vi "LightSheet_Example_IMAQ.vi"() -> ()   [LabVIEW 2019]
doc: "This example is similar to the simple example, but uses get/set line timeing for controlling the exposure.\nExposureTime = LineTime * ExposureLines\nBeside of the line timing part, a simple recording of an image sequence and the image access afterwards is done.\nIt is a good starting point for writing own applications, especially for light sheet application development.\nBut it will not be fail save, i.e. doesnt react on errors, just handles them forward to the end\n\nUsage:\nSelect your required image count and the required line tiime + number of exposure lines before you start the program.\nOnce started, the camera class will be initialized and images will be recorded automatically.\nWhen acquisition has finished you can address the images and set a certain roi \nTo finish the program click on quit application, this will force fan exit of the camera class"
uses:
  camera/Camera.lvclass
  pco.sdk/SpecialCommandsEdge/SpecialCommandsEdge.lvlib
panel:
  in  "dwExposureLines":u32=100
  in  "wTimeBase":u16(ring)=1 items=["ns", "us", "ms"]
  in  "dwLineTime":u32=50
  out "rawImage":u16[][](array[numeric])
  out "Image":T1(plugin-control)
  in  "data_format":T2(ring)=enum."Mono16"
  in  "Image Index":u32 max=99
  out "Recorded Images":u32
  in  "Quit":bool
  in  "cropY1":u64=2 min=2 max=1040 step=1
  in  "cropX1":u64=2 min=2 max=1392 step=1
  in  "cropY0":u64=1 min=1 max=1039 step=1
  in  "cropX0":u64=1 min=1 max=1391 step=1
  out "Image Height":u64
  out "Image Width":u64
  in  "dwImgCount":u32=10 caption="Required Number of Images" max=4023
  out "Error":errorcluster {"code" format="%x"}
  # "This example is similar to the simple example, but uses get/set line timeing for controlling the exposure.\nExposureTime = LineTime * ExposureLines\nBeside of the line timing part, a simple recording of an image sequence and the image access afterwards is done.\nIt is a good starting point for writing own applications, especially  for light sheet application development.\nBut it will not be fail save, i.e. doesnt react on errors, just handles them forward to the end\n\nUsage:\nSelect your required image count and the required line tiime + number of exposure lines before you start the program.\nOnce started, the camera class will be initialized and images will be recorded automatically.\nWhen acquisition has finished you can address the images and set a certain roi \nTo finish the program click on quit application, this will force fan exit of the camera class"
  # "pco.labview"
  # "Camera Setup"
  # "Recording Control"
  # "Parameters for image readout"
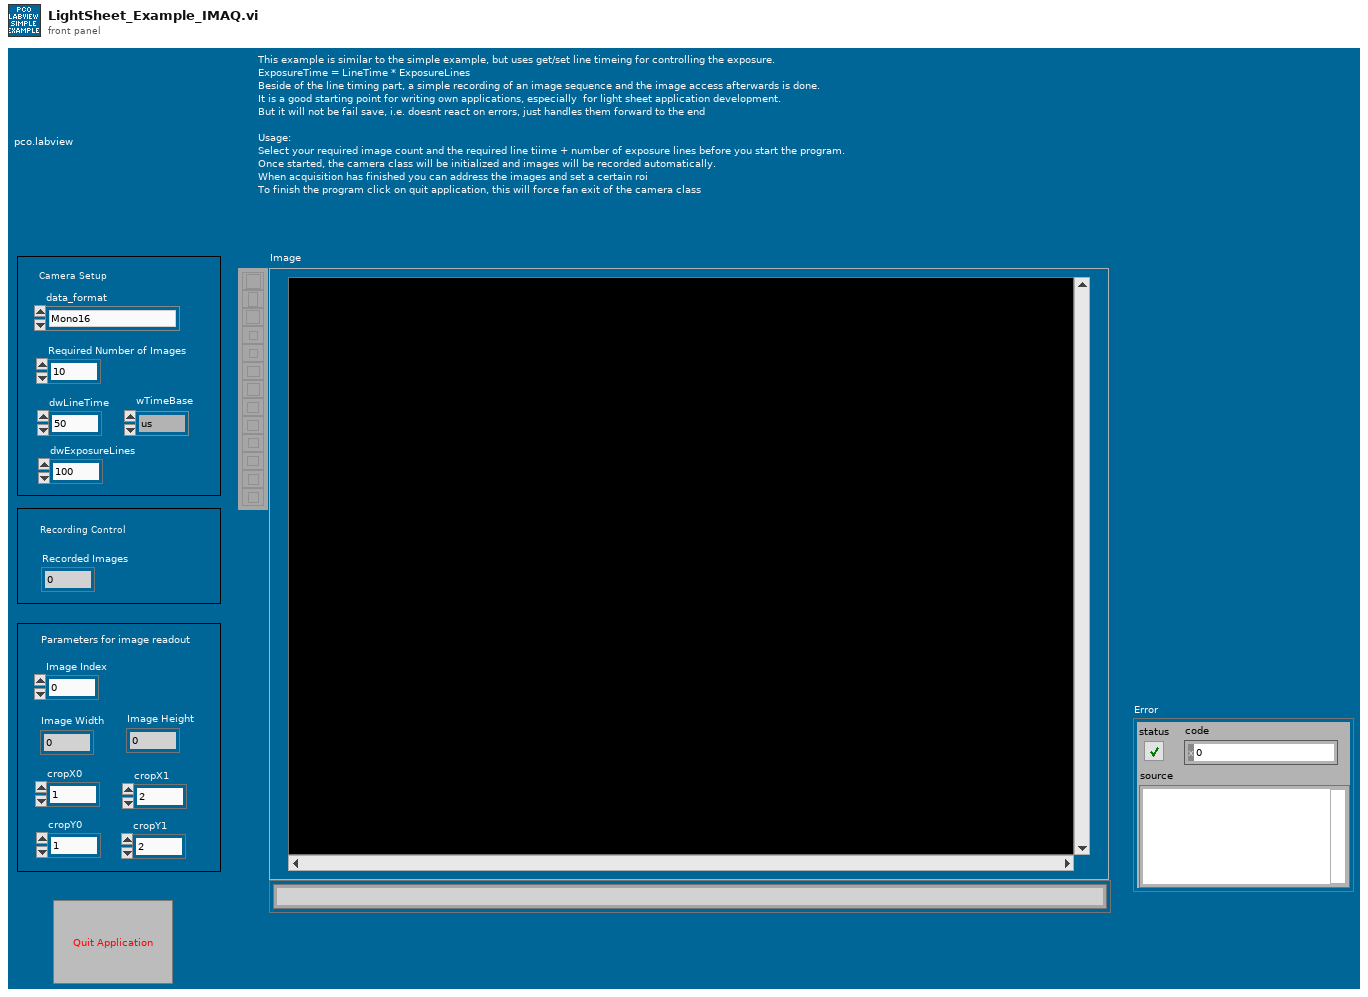
[diagram p1: front panel]
types:
  T1 = typedef "IMAQ Image.ctl" = refnum<image>
  T2 = enum16{"Undefined", "Mono8", "Mono16", "BGRA8", "RGBA8", "BGRA16", "RGBA16", "CompressedMono8"}
  T3 = enum8{"Enabled", "Disabled", "Disabled and Grayed Out"}
  T4 = enum16{"sequence", "sequence non blocking", "ring buffer", "fifo", "tif", "multitif", "pcoraw", "b16", "dicom", "multidicom", "camram_ring", "camram_segment"}
  T5 = cluster{"serial":u32, "type":u16, "sub_type":u16, "interface_type":u16, "bit_resolution":u16, "min_exposure_time_s":dbl, "max_exposure_time_s":dbl, "min_exposure_step_s":dbl, "min_delay_time_s":dbl, "max_delay_time_s":dbl, "min_delay_step_s":dbl, "min_width":u64, "min_height":u64, "max_width":u64, "max_height":u64, "roi_step_horz":u64, "roi_step_vert":u64, "roi_symmetric_horz":bool, "roi_symmetric_vert":bool, "has_timestamp_mode":bool, "has_timestamp_mode_ascii_only":bool, "pixelrate_vec":u32[], "conversion_factor_vec":sgl[], "has_trigger_mode_extexpctrl":bool, "has_acquire_mode":bool, "has_ext_acquire_mode":bool, "has_metadata_mode":bool, "has_ram":bool, "binning_horz_vec":u16[], "binning_vert_vec":u16[], "has_average_binning":bool, "pixel_format_vec":u32[]}
  T6 = typedef "Image Type" = u32
  T7 = typedef "Camera.lvclass/binning.ctl" = cluster{"vert":u16, "horz":u16, "mode":u16}
  T8 = cluster{"exposure_time_s":dbl, "delay_time_s":dbl, "roi":cluster{"x0":u64, "y0":u64, "x1":u64, "y1":u64}, "timestamp_mode":u16, "pixelrate":u32, "conversion_factor":sgl, "trigger_mode":u16, "acquire_mode":u16, "acquire_sequence_number":u32, "metadata_mode":u16, "noisefilter_mode":u16, "pixel_format":u32, "binning":T7, "auto_exposure":cluster{"region":u16, "min_exposure_s":dbl, "max_exposure_s":dbl}}
  T9 = cluster{"Plane 4 (alpha)":u16, "Plane 1 (Red)":u16, "Plane 2 (Green)":u16, "Plane 3 (Blue)":u16}[][]
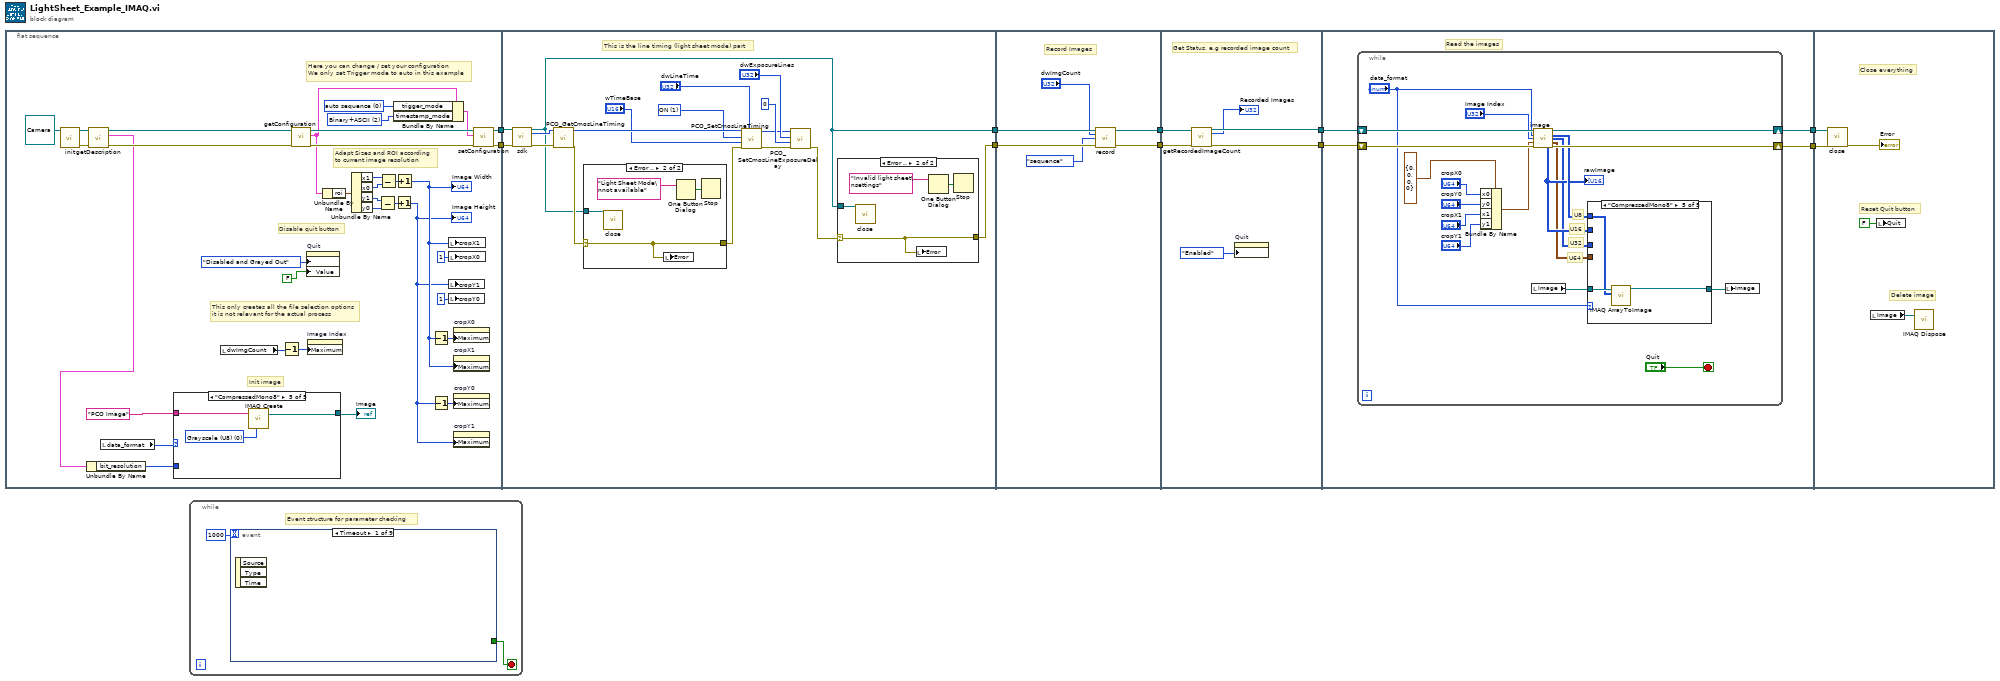
[diagram p0: block diagram]
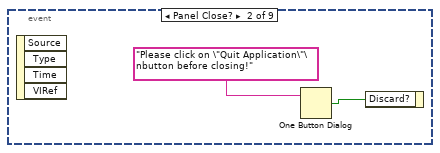
[diagram p2: hidden frame]
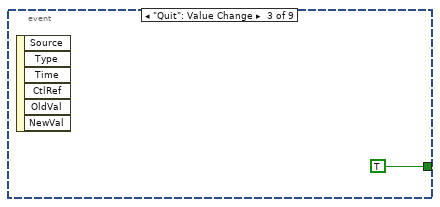
[diagram p3: hidden frame]
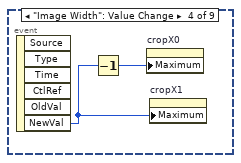
[diagram p4: hidden frame]
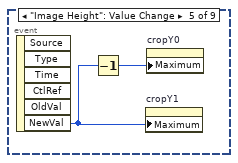
[diagram p5: hidden frame]
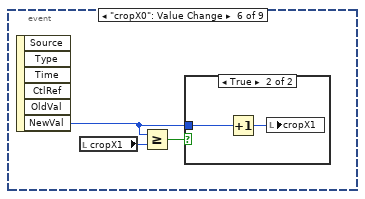
[diagram p6: hidden frame]
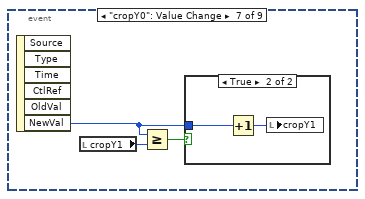
[diagram p8: hidden frame]
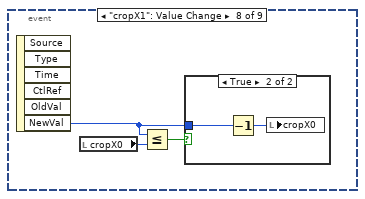
[diagram p10: hidden frame]
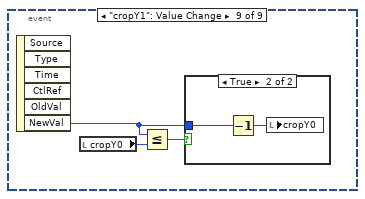
[diagram p12: hidden frame]
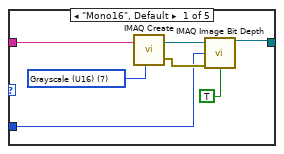
[diagram p14: hidden frame]
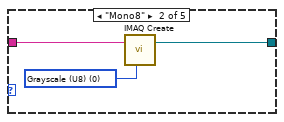
[diagram p15: hidden frame]
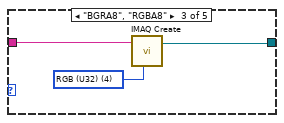
[diagram p16: hidden frame]
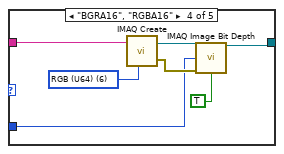
[diagram p17: hidden frame]
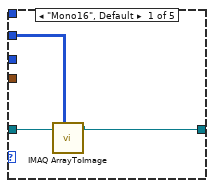
[diagram p20: hidden frame]
diagram:
  n1 = flat-sequence {
    tunnel: [w40] -> w4
    tunnel: [w39] -> w2
    tunnel: w4 -> [w81]
    tunnel: [w69] -> w3
    tunnel: w2 -> [w80]
    tunnel: [w70] -> w1
    tunnel: w3 -> [w101]
    tunnel: w1 -> [w100]
    tunnel: [w98] -> w10
    tunnel: [w97] -> w9
    tunnel: w10 -> [w107]
    tunnel: w9 -> [w106]
    tunnel: [w105] -> w8
    tunnel: [w104] -> w7
    tunnel: w8 -> [w110]
    tunnel: w7 -> [w111]
    tunnel: [w109] -> w6
    tunnel: [w108] -> w5
    tunnel: w6 -> [w148]
    tunnel: w5 -> [w147]
    frame #0 {
      w24 = u16 2 items=["OFF", "Binary", "Binary+ASCII", "ASCII"] ("TimestampMode")
      w44 = u16 0 items=["auto sequence"=0, "software trigger"=1, "external exposure start & software trigger"=2, "external exposure control"=3, "external synchronized"=4, "fast external exposure control"=5, "external CDS control"=6, "slow external exposure control"=7, "external synchronized HDSDI"=258] ("TriggerMode")
      # "Init image"
      # "This only creates all the file selection options\nit is not relevant for the actual process"
      # "Adapt Sizes and ROI according\nto current image resolution"
      # "Disable quit button"
      # "Here you can change / set your configuration\nWe only set Trigger mode to auto in this example"
      n2 = call-dynamic "init.vi"("Camera in"=refnum<class "Camera.lvclass"> refnum ("PCOCamera in")) -> ("Camera out"=w15:refnum<class "Camera.lvclass">, "error out"=w16:errorcluster)  [unwired: 8 in]
      n3 = call-dynamic "getDescription.vi"("error in (no error)"=w16, "Camera in"=w15) -> ("error out"=w13:errorcluster, "description"=w12:T5, "Camera out"=w14:refnum<class "Camera.lvclass">)  [unwired: 7 in]
      n4 = Unbundle By Name(w12) -> ("bit_resolution"=w11:u16)
      n5 = local read "data_format"() -> (w19:T2)
      n6 = case shown="\"CompressedMono8\"" w19 {
        tunnel: "PCO Image" ("Image Name") -> [w51 w55 w57 w64 w67]
        tunnel: [w47 w53 w56 w61 w66] -> w18
        tunnel: w11 -> [w46 _ _ w59 _]
        frame "Mono16", Default {
          w52 = T6 7 items=["Grayscale (U8)", "Grayscale (I16)", "Grayscale (SGL)", "Complex (CSG)", "RGB (U32)", "HSL (U32)", "RGB (U64)", "Grayscale (U16)"] ("Image Type")
          n7 = call "IMAQ Create"("Image Name"=w51, "Image Type"=w52) -> ("New Image"=w49:T1, "error out"=w48:errorcluster)  [unwired: 3 in]
          n8 = call "IMAQ Image Bit Depth"("Image"=w49, "Bit Depth (0)"=w46, "error in (no error)"=w48, "Get/Set Bit Depth? (Set)"=TRUE) -> ("Image Out"=w47:T1)  [unwired: 9 in, 2 out]
        }
        frame "Mono8" {
          w54 = T6 0 items=["Grayscale (U8)", "Grayscale (I16)", "Grayscale (SGL)", "Complex (CSG)", "RGB (U32)", "HSL (U32)", "RGB (U64)", "Grayscale (U16)"] ("Image Type")
          n9 = call "IMAQ Create"("Image Name"=w55, "Image Type"=w54) -> ("New Image"=w53:T1)  [unwired: 3 in, 1 out]
        }
        frame "BGRA8", "RGBA8" {
          w58 = T6 4 items=["Grayscale (U8)", "Grayscale (I16)", "Grayscale (SGL)", "Complex (CSG)", "RGB (U32)", "HSL (U32)", "RGB (U64)", "Grayscale (U16)"] ("Image Type")
          n10 = call "IMAQ Create"("Image Name"=w57, "Image Type"=w58) -> ("New Image"=w56:T1)  [unwired: 3 in, 1 out]
        }
        frame "BGRA16", "RGBA16" {
          w65 = T6 6 items=["Grayscale (U8)", "Grayscale (I16)", "Grayscale (SGL)", "Complex (CSG)", "RGB (U32)", "HSL (U32)", "RGB (U64)", "Grayscale (U16)"] ("Image Type")
          n11 = call "IMAQ Create"("Image Name"=w64, "Image Type"=w65) -> ("New Image"=w62:T1, "error out"=w60:errorcluster)  [unwired: 3 in]
          n12 = call "IMAQ Image Bit Depth"("Image"=w62, "Bit Depth (0)"=w59, "error in (no error)"=w60, "Get/Set Bit Depth? (Set)"=TRUE) -> ("Image Out"=w61:T1)  [unwired: 9 in, 2 out]
        }
        frame "CompressedMono8" {
          w68 = T6 0 items=["Grayscale (U8)", "Grayscale (I16)", "Grayscale (SGL)", "Complex (CSG)", "RGB (U32)", "HSL (U32)", "RGB (U64)", "Grayscale (U16)"] ("Image Type")
          n13 = call "IMAQ Create"("Image Name"=w67, "Image Type"=w68) -> ("New Image"=w66:T1)  [unwired: 3 in, 1 out]
        }
      }
      "Image" <- w18
      n14 = local read "dwImgCount"() -> (w20:u32)
      n15 = Decrement(x=w20) -> (x-1=w21:u32)
      n16 = call-dynamic "getConfiguration.vi"("error in (no error)"=w13, "Camera in"=w14) -> ("error out"=w42:errorcluster, "configuration"=w34:T8, "Camera out"=w43:refnum<class "Camera.lvclass">)  [unwired: 7 in]
      n17 = property on="Quit" class="Bool (strict)"("DisabledEnum"=T3."Disabled and Grayed Out" ("Disabled"), "Value"=FALSE ("Stop")) -> ()  [unwired: 2 in, 2 out]
      n18 = property on="Image Index" class="DigNum (strict)"("Maximum"=w21) -> ()  [unwired: 2 in, 2 out]
      n19 = Unbundle By Name(w34) -> ("roi"=w33:cluster{"x0":u64, "y0":u64, "x1":u64, "y1":u64})
      n20 = Unbundle By Name(w33) -> ("x1"=w31:u64, "x0"=w32:u64, "y1"=w29:u64, "y0"=w30:u64)
      n21 = Subtract(x=w29, y=w30) -> (x-y=w27:u64)
      n22 = Subtract(x=w31, y=w32) -> (x-y=w28:u64)
      n23 = Bundle By Name(cluster=w34, "trigger_mode"=w44, "timestamp_mode"=w24) -> (w41:T8)
      n24 = Increment(x=w27) -> (x+1=w25:u64)
      "Image Height" <- w25
      n25 = Increment(x=w28) -> (x+1=w26:u64)
      "Image Width" <- w26
      n26 = Decrement(x=w26) -> (x-1=w36:u64)
      n27 = Decrement(x=w25) -> (x-1=w35:u64)
      n28 = local write "cropX1"(w26) -> ()
      n29 = local write "cropX0"(u64 1 ("roiY0")) -> ()
      n30 = local write "cropY1"(w25) -> ()
      n31 = local write "cropY0"(u64 1 ("roiY0")) -> ()
      n32 = property on="cropX0" class="DigNum (strict)"("Maximum"=w36) -> ()  [unwired: 2 in, 2 out]
      n33 = property on="cropX1" class="DigNum (strict)"("Maximum"=w26) -> ()  [unwired: 2 in, 2 out]
      n34 = property on="cropY0" class="DigNum (strict)"("Maximum"=w35) -> ()  [unwired: 2 in, 2 out]
      n35 = property on="cropY1" class="DigNum (strict)"("Maximum"=w25) -> ()  [unwired: 2 in, 2 out]
      n36 = call-dynamic "setConfiguration.vi"("error in (no error)"=w42, "configuration"=w41, "Camera in"=w43) -> ("error out"=w39:errorcluster, "Camera out"=w40:refnum<class "Camera.lvclass">)  [unwired: 7 in]
    }
    frame #1 {
      w77 = u16 1 items=["OFF", "ON"] ("wParameter")
      # "This is the line timing (light sheet mode) part"
      n37 = call-dynamic "sdk.vi"("Camera in"=w81, "error in (no error)"=w80) -> ("Camera out"=w69:refnum<class "Camera.lvclass">, "sdk"=w79:u64, "error out"=w85:errorcluster)  [unwired: 11 in]
      n38 = call "PCO_GetCmosLineTiming.vi"("ph"=w79, "error in (no error)"=w85) -> ("ph out"=w78:u64, "error out"=w84:errorcluster)  [unwired: 10 in, 6 out]
      n39 = case shown="Error .." w84 {
        selector: w84 -> [w91 w92]
        tunnel: [w91 w92] -> w83
        tunnel: w69 -> [_ w93]
        frame No Error {
        }
        frame Error {
          n40 = call-dynamic "close.vi"("Camera in"=w93) -> ()  [unwired: 10 in, 1 out]
          n41 = local write "Error"(w92) -> ()
          n42 = One Button Dialog(message="Light Sheet Mode\nnot available") -> (true=w94:bool)  [unwired: 1 in]
          n43 = Stop(stop? (T)=w94) -> ()
        }
      }
      n44 = call "PCO_SetCmosLineTiming.vi"("dwLineTime"="dwLineTime", "error in (no error)"=w83, "wTimeBase"="wTimeBase", "wParameter"=w77, "ph"=w78) -> ("error out"=w82:errorcluster, "ph out"=w72:u64)  [unwired: 4 in, 1 out]
      n45 = call "PCO_SetCmosLineExposureDelay.vi"("error in (no error)"=w82, "dwDelayLines"=u32 0, "dwExposureLines"="dwExposureLines", "ph"=w72) -> ("error out"=w71:errorcluster)  [unwired: 5 in, 2 out]
      n46 = case shown="Error .." w71 {
        selector: w71 -> [w86 w87]
        tunnel: [w86 w87] -> w70
        tunnel: w69 -> [_ w88]
        frame No Error {
        }
        frame Error {
          n47 = call-dynamic "close.vi"("Camera in"=w88) -> ()  [unwired: 10 in, 1 out]
          n48 = local write "Error"(w87) -> ()
          n49 = One Button Dialog(message="Invalid light sheet\nsettings") -> (true=w89:bool)  [unwired: 1 in]
          n50 = Stop(stop? (T)=w89) -> ()
        }
      }
    }
    frame #2 {
      # "Record Images"
      n51 = call-dynamic "record.vi"("Camera in"=w101, "num_images"="dwImgCount", "record_mode"=T4."sequence", "error in (no error)"=w100) -> ("Camera out"=w98:refnum<class "Camera.lvclass">, "error out"=w97:errorcluster)  [unwired: 10 in]
    }
    frame #3 {
      # "Get Status, e.g recorded image count"
      n52 = call-dynamic "getRecordedImageCount.vi"("Camera in"=w107, "error in (no error)"=w106) -> ("Camera out"=w105:refnum<class "Camera.lvclass">, "recorded_image_count"=→"Recorded Images":u32, "error out"=w104:errorcluster)  [unwired: 11 in]
      n53 = property on="Quit" class="Bool (strict)"("DisabledEnum"=T3."Enabled" ("Disabled")) -> ()  [unwired: 2 in, 2 out]
    }
    frame #4 {
      # "Read the images"
      n54 = while {
        shift-right: [w128] -> w109
        shift-left: w110 -> [w130]
        shift-right: [w123] -> w108
        shift-left: w111 -> [w129]
        stop <- "Quit" stop-if-true
        # "U64"
        # "U32"
        # "U16"
        # "U8"
        n55 = Bundle By Name(cluster=cluster{"x0":u64, "y0":u64, "x1":u64, "y1":u64} {"x0"=0, "y0"=0, "x1"=0, "y1"=0} ("roi"), "x0"="cropX0", "y0"="cropY0", "x1"="cropX1", "y1"="cropY1") -> (w122:cluster{"x0":u64, "y0":u64, "x1":u64, "y1":u64})
        n56 = local read "Image"() -> (w115:T1)
        n57 = call-dynamic "image.vi"("Camera in"=w130, "data_format"="data_format", "image_index"="Image Index", "crop"=w122, "error in (no error)"=w129) -> ("Camera out"=w128:refnum<class "Camera.lvclass">, "image (U8)"=w119:u8[][], "image (U32)"=w117:u32[][], "image (U64)"=w116:T9, "raw_image (U16)"=w118:u16[][], "error out"=w123:errorcluster)  [unwired: 2 in, 3 out]
        "rawImage" <- w118
        n58 = case shown="\"CompressedMono8\"" "data_format" {
          tunnel: w115 -> [w133 w136 w139 w142 w145]
          tunnel: [w131 w134 w138 w140 w144] -> w114
          tunnel: w116 -> [_ _ _ w141 _]
          tunnel: w117 -> [_ _ w137 _ _]
          tunnel: w119 -> [_ w135 _ _ w143]
          tunnel: w118 -> [w132 _ _ _ _]
          frame "Mono16", Default {
            n59 = call "IMAQ ArrayToImage"("Image Pixels (U16)"=w132, "Image"=w133) -> ("Image Out"=w131:T1)  [unwired: 8 in, 1 out]
          }
          frame "Mono8" {
            n60 = call "IMAQ ArrayToImage"("Image Pixels (U8)"=w135, "Image"=w136) -> ("Image Out"=w134:T1)  [unwired: 8 in, 1 out]
          }
          frame "BGRA8", "RGBA8" {
            n61 = call "IMAQ ArrayToColorImage"("Image Pixels (U32)"=w137, "Image"=w139) -> ("Image Out"=w138:T1)  [unwired: 3 in, 1 out]
          }
          frame "BGRA16", "RGBA16" {
            n62 = call "IMAQ ArrayToColorImage"("Image"=w142, "Image Pixels (U64)"=w141) -> ("Image Out"=w140:T1)  [unwired: 3 in, 1 out]
          }
          frame "CompressedMono8" {
            n63 = call "IMAQ ArrayToImage"("Image Pixels (U8)"=w143, "Image"=w145) -> ("Image Out"=w144:T1)  [unwired: 8 in, 1 out]
          }
        }
        n64 = local write "Image"(w114) -> ()
      }
    }
    frame #5 {
      # "Delete image"
      # "Reset Quit button"
      # "Close everything"
      n65 = call-dynamic "close.vi"("error in (no error)"=w147, "Camera in"=w148) -> ("error out"=→"Error":errorcluster)  [unwired: 9 in]
      n66 = local read "Image"() -> (w146:T1)
      n67 = local write "Quit"(FALSE ("Stop")) -> ()
      n68 = call "IMAQ Dispose"("Image"=w146) -> ()  [unwired: 5 in, 1 out]
    }
  }
  n69 = while {
    stop <- w151 stop-if-true
    # "Event structure for parameter checking"
    n70 = event shown="[0] Timeout" {
      selector: _ -> [_ _ _ _ _ _ _ _ _]
      dyn-events: _ -> [_ _ _ _ _ _ _ _ _]
      timeout: 1000 -> [_ _ _ _ _ _ _ _ _]
      tunnel: [_ _ TRUE _ _ _ _ _ _] -> w151
      event Timeout {
        n71 = event-data() -> ()  [unwired: 1 in, 3 out]
      }
      event Panel Close? {
        n72 = event-data() -> ()  [unwired: 1 in, 4 out]
        n73 = One Button Dialog(message="Please click on \"Quit Application\"\nbutton before closing!") -> (true=w153:bool)  [unwired: 1 in]
        n74 = event-data("Discard?"=w153) -> ()  [unwired: 1 in, 1 out]
      }
      event "Quit": Value Change {
        n75 = event-data() -> ()  [unwired: 1 in, 6 out]
      }
      event "Image Width": Value Change {
        n76 = event-data() -> ("NewVal"=w156:u64)  [unwired: 1 in, 5 out]
        n77 = Decrement(x=w156) -> (x-1=w157:u64)
        n78 = property on="cropX0" class="DigNum (strict)"("Maximum"=w157) -> ()  [unwired: 2 in, 2 out]
        n79 = property on="cropX1" class="DigNum (strict)"("Maximum"=w156) -> ()  [unwired: 2 in, 2 out]
      }
      event "Image Height": Value Change {
        n80 = event-data() -> ("NewVal"=w158:u64)  [unwired: 1 in, 5 out]
        n81 = Decrement(x=w158) -> (x-1=w159:u64)
        n82 = property on="cropY1" class="DigNum (strict)"("Maximum"=w158) -> ()  [unwired: 2 in, 2 out]
        n83 = property on="cropY0" class="DigNum (strict)"("Maximum"=w159) -> ()  [unwired: 2 in, 2 out]
      }
      event "cropX0": Value Change {
        n84 = event-data() -> ("NewVal"=w160:u64)  [unwired: 1 in, 5 out]
        n85 = local read "cropX1"() -> (w162:u64)
        n86 = Greater Or Equal?(x=w160, y=w162) -> (x >= y?=w161:bool)
        n87 = case shown="True" w161 {
          tunnel: w160 -> [_ w164]
          frame False {
          }
          frame True {
            n88 = Increment(x=w164) -> (x+1=w163:u64)
            n89 = local write "cropX1"(w163) -> ()
          }
        }
      }
      event "cropY0": Value Change {
        n90 = event-data() -> ("NewVal"=w165:u64)  [unwired: 1 in, 5 out]
        n91 = local read "cropY1"() -> (w167:u64)
        n92 = Greater Or Equal?(x=w165, y=w167) -> (x >= y?=w166:bool)
        n93 = case shown="True" w166 {
          tunnel: w165 -> [_ w169]
          frame False {
          }
          frame True {
            n94 = Increment(x=w169) -> (x+1=w168:u64)
            n95 = local write "cropY1"(w168) -> ()
          }
        }
      }
      event "cropX1": Value Change {
        n96 = event-data() -> ("NewVal"=w170:u64)  [unwired: 1 in, 5 out]
        n97 = local read "cropX0"() -> (w172:u64)
        n98 = Less Or Equal?(x=w170, y=w172) -> (x <= y?=w171:bool)
        n99 = case shown="True" w171 {
          tunnel: w170 -> [_ w174]
          frame False {
          }
          frame True {
            n100 = Decrement(x=w174) -> (x-1=w173:u64)
            n101 = local write "cropX0"(w173) -> ()
          }
        }
      }
      event "cropY1": Value Change {
        n102 = event-data() -> ("NewVal"=w175:u64)  [unwired: 1 in, 5 out]
        n103 = local read "cropY0"() -> (w177:u64)
        n104 = Less Or Equal?(x=w175, y=w177) -> (x <= y?=w176:bool)
        n105 = case shown="True" w176 {
          tunnel: w175 -> [_ w179]
          frame False {
          }
          frame True {
            n106 = Decrement(x=w179) -> (x-1=w178:u64)
            n107 = local write "cropY0"(w178) -> ()
          }
        }
      }
    }
  }
